vi "RenamePropertyMethods.vi"(10 "RenameToGet/Set":bool, 11 "PropertyNodeMethods":T1[](array[typedef])) -> (3 "Array":T1[](array[typedef]))   [LabVIEW 2020, in "ClassWriterNative.lvclass"]
uses:
  ClassWriterNative.lvclass
  MethodInfo.ctl
  MethodType.ctl
  MethodInfo_Option.ctl
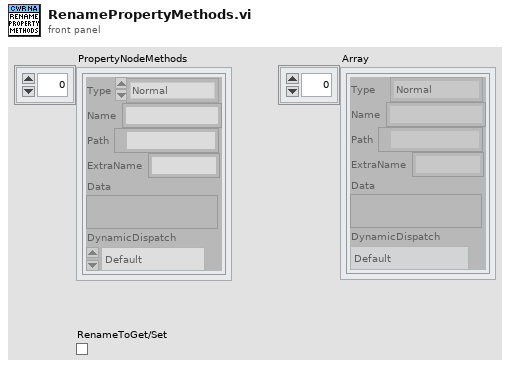
[diagram p1: front panel]
types:
  T1 = typedef "ClassWriterNative.lvclass/MethodInfo.ctl" = cluster{"Type":T2, "Name":string, "Path":path, "ExtraName":string, "Data":variant, "DynamicDispatch":T3}
  T2 = typedef "ClassWriterNative.lvclass/MethodType.ctl" = enum16{"Normal", "MethodPlugIn", "DesignPattern", "AF-Method"}
  T3 = typedef "ClassWriterNative.lvclass/MethodInfo_Option.ctl" = enum16{"Default", "OnAtStart", "OffAtStart", "AlwaysOn", "AlwaysOff"}
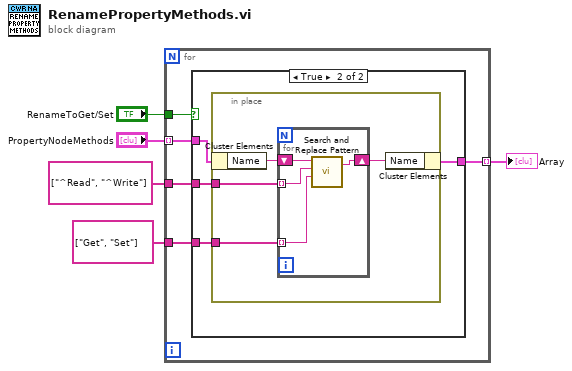
[diagram p0: block diagram]
diagram:
  n1 = for {
    tunnel: "PropertyNodeMethods" -> [w10] mode=indexing
    tunnel: "RenameToGet/Set" -> [w9]
    tunnel: string[] ["^Read", "^Write"] ("regular expression (\"\")") -> [w8]
    tunnel: string[] ["Get", "Set"] ("regular expression (\"\")") -> [w7]
    tunnel: [w6] -> w5 mode=indexing
    n2 = case shown="True" w9 {
      tunnel: w10 -> [w11 w15]
      tunnel: w8 -> [_ w14]
      tunnel: w7 -> [_ w13]
      tunnel: [w11 w12] -> w6
      frame False {
      }
      frame True {
        n3 = in-place {
          in-place-border: w14 -> [w17]
          in-place-border: w13 -> [w16]
          n4 = in-place-cluster #1(w15) -> ("Name"=w19:string)
          n5 = for {
            tunnel: w17 -> [w21] mode=indexing
            tunnel: w16 -> [w20] mode=indexing
            shift-right: [w22] -> w18
            shift-left: w19 -> [w23]
            n6 = call <vilib>:"Search and Replace Pattern.vi"("string"=w23, "regular expression (\"\")"=w21, "replace string (\"\")"=w20) -> ("result string"=w22:string)  [unwired: 2 in, 1 out]
          }
          n7 = in-place-cluster #1("Name"=w18) -> (w12:T1)
        }
      }
    }
  }
  "Array" <- w5
